vi "test_Create directory.vi"(8 "error in (no error)":errorcluster, 11 "TestCase in":refnum<class "[Test Case] Create directory.lvclass">) -> (0 "error out":errorcluster, 3 "TestCase out":refnum<class "[Test Case] Create directory.lvclass">)   [LabVIEW 2015, in "Tests.lvlib" / "[Test Case] Create directory.lvclass"]
uses:
  [Test Case] Create directory.lvclass
  [Test Case] Create directory.lvclass/[Test Case] Create directory.ctl
  classes/File Transfer Behavior/File Transfer Behavior.lvclass
  <vilib>/addons/_JKI Toolkits/VI Tester/TestCase.llb/TestCase.lvclass
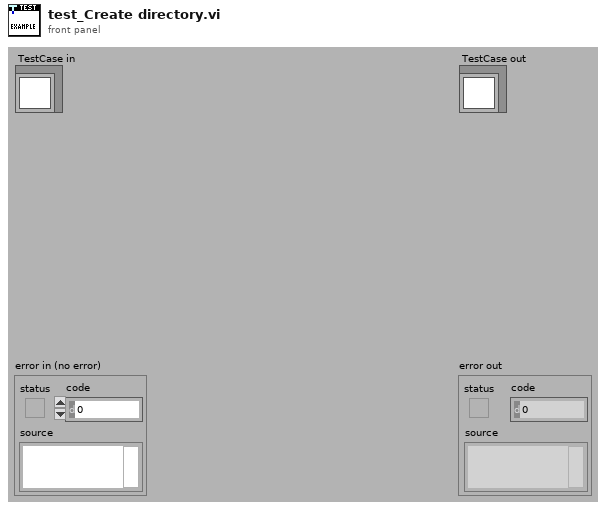
[diagram p1: front panel]
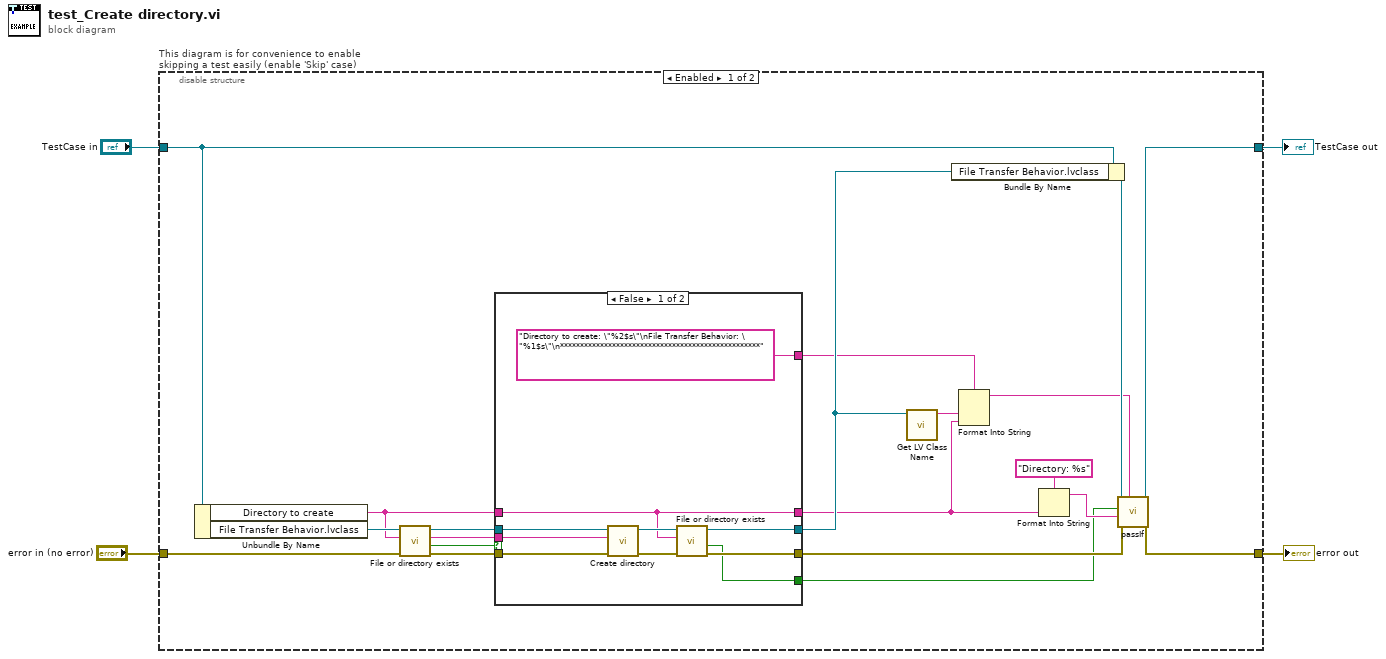
[diagram p0: block diagram]
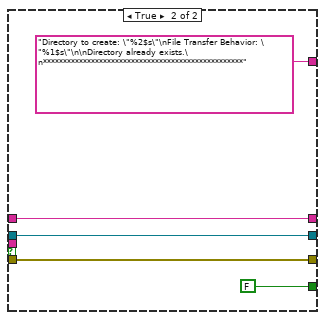
[diagram p2: hidden frame]
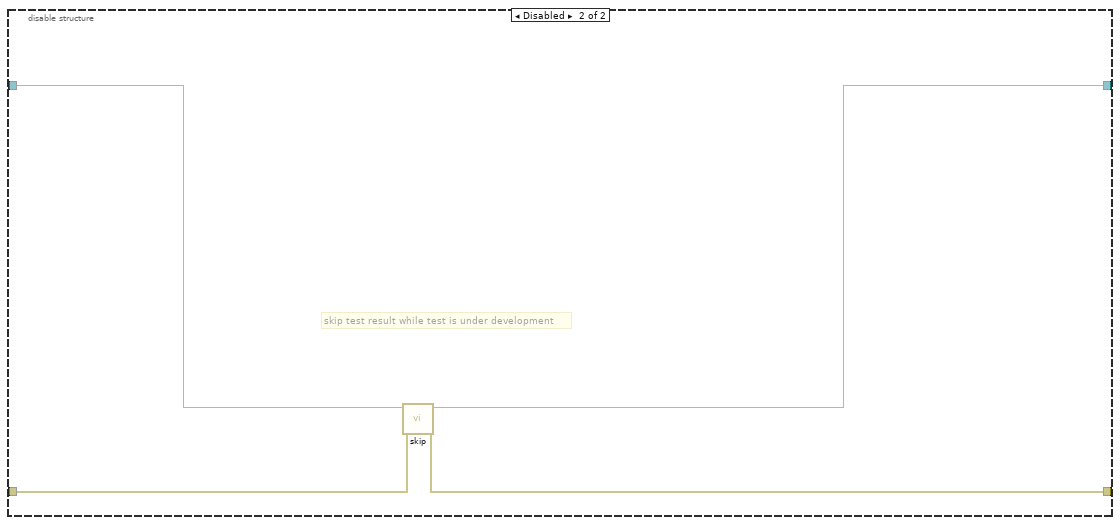
[diagram p3: hidden frame]
diagram:
  n1 = disable-structure "This diagram is for convenience to enable skipping a test easily (enable 'Skip' case)" shown="Enabled" {
    disable-tunnel: "TestCase in" -> [w21 w43]
    disable-tunnel: [w24 w41] -> w1
    disable-tunnel: [w23 w42] -> w3
    disable-tunnel: "error in (no error)" -> [w15 w40]
    frame Enabled {
      n2 = Unbundle By Name(w21) -> ("Directory to create"=w10:string, "File Transfer Behavior.lvclass"=w16:refnum<class "File Transfer Behavior.lvclass">)
      n3 = call-dynamic "File or directory exists.vi"("error in (no error)"=w15, "Path"=w10, "File Transfer Behavior in"=w16) -> ("error out"=w18:errorcluster, "Exists?"=w8:bool, "Path out (dup)"=w14:string, "File Transfer Behavior out"=w17:refnum<class "File Transfer Behavior.lvclass">)  [unwired: 4 in, 1 out]
      n4 = case shown="False" w8 {
        tunnel: [w32 w38] -> w22
        tunnel: w18 -> [w31 w38]
        tunnel: w17 -> [w30 w39]
        tunnel: w14 -> [w29 _]
        tunnel: [w28 w39] -> w12
        tunnel: w10 -> [w27 w37]
        tunnel: [w27 w37] -> w7
        tunnel: [w26 FALSE] -> w6
        tunnel: ["Directory to create: \"%2$s\"\nFile Transfer Behavior: \"%1$s\"\n**************************************************" ("format string") "Directory to create: \"%2$s\"\nFile Transfer Behavior: \"%1$s\"\n\nDirectory already exists.\n**************************************************" ("format string")] -> w5
        frame False {
          n5 = call-dynamic "Create directory.vi"("error in (no error)"=w31, "Directory"=w29, "File Transfer Behavior in"=w30) -> ("error out"=w33:errorcluster, "File Transfer Behavior out"=w34:refnum<class "File Transfer Behavior.lvclass">)  [unwired: 7 in]
          n6 = call-dynamic "File or directory exists.vi"("error in (no error)"=w33, "Path"=w27, "File Transfer Behavior in"=w34) -> ("error out"=w32:errorcluster, "Exists?"=w26:bool, "File Transfer Behavior out"=w28:refnum<class "File Transfer Behavior.lvclass">)  [unwired: 4 in, 2 out]
        }
        frame True {
        }
      }
      n7 = call <vilib>:"Get LV Class Name.vi"("object"=w12) -> ("class name"=w11:string)  [unwired: 9 in, 1 out]
      n8 = Bundle By Name(cluster=w21, "File Transfer Behavior.lvclass"=w12) -> (w20:refnum<class "[Test Case] Create directory.lvclass">)
      n9 = Format Into String(format string=w5, w11, w7) -> (resulting string=w9:string)  [unwired: 2 in, 1 out]
      n10 = Format Into String(format string="Directory: %s", w7) -> (resulting string=w13:string)  [unwired: 2 in, 1 out]
      n11 = call-dynamic "passIf.vi"("custom report message (\"\")"=w9, "error in (no error)"=w22, "message (\"\")"=w13, "pass"=w6, "TestCase in"=w20) -> ("error out"=w23:errorcluster, "TestCase out"=w24:refnum<class "[Test Case] Create directory.lvclass">)  [unwired: 5 in]
    }
    frame Disabled {
      # "skip test result while test is under development"
      n12 = call <vilib>:"skip.vi"("error in (no error)"=w40, "TestCase in"=w43) -> ("error out"=w42:errorcluster, "TestCase out"=w41:refnum<class "[Test Case] Create directory.lvclass">)  [unwired: 8 in]
    }
  }
  "error out" <- w3
  "TestCase out" <- w1
